vi "estiOptState.vi"(7 "Filter Type":u16(ring) items=["ref", "u", "g", "r", "i", "z", "y"], 8 "error in (no error)":errorcluster, 9 "Field Idx":i32[](array[numeric]), 10 "Zk":dbl[][](array[numeric]), 11 "OptStateEsti in":refnum<class "OptStateEsti.lvclass">) -> (0 "error out":errorcluster, 2 "Optical State":dbl[](array[numeric]), 3 "OptStateEsti out":refnum<class "OptStateEsti.lvclass">)   [LabVIEW 2016, in "OptStateEsti.lvclass"]
doc: "Estimate the optical state in the basis of degree of freedom (DOF)."
uses:
  OptStateEsti.lvclass
  OptStateEsti.lvclass/OptStateEsti.ctl
  <vilib>/Analysis/baseanly.llb/Real A x B.vi
  Utility/getSubArray2D.vi
  <vilib>/Analysis/Matrix/Numeric/Conversions/Array To Matrix - RA2.vi
  <vilib>/Analysis/Matrix/Numeric/Conversions/Matrix To Array - RM.vi
  <vilib>/Analysis/Matrix/NI_Matrix.lvlib
  <vilib>/Analysis/NI_AALBase.lvlib
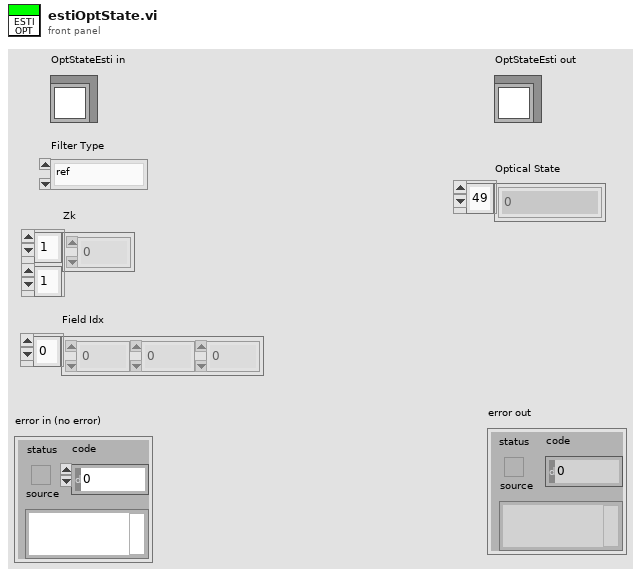
[diagram p1: front panel]
types:
  T1 = typedef "NI_Matrix.lvlib/RealMatrix.ctl" = dbl[][]
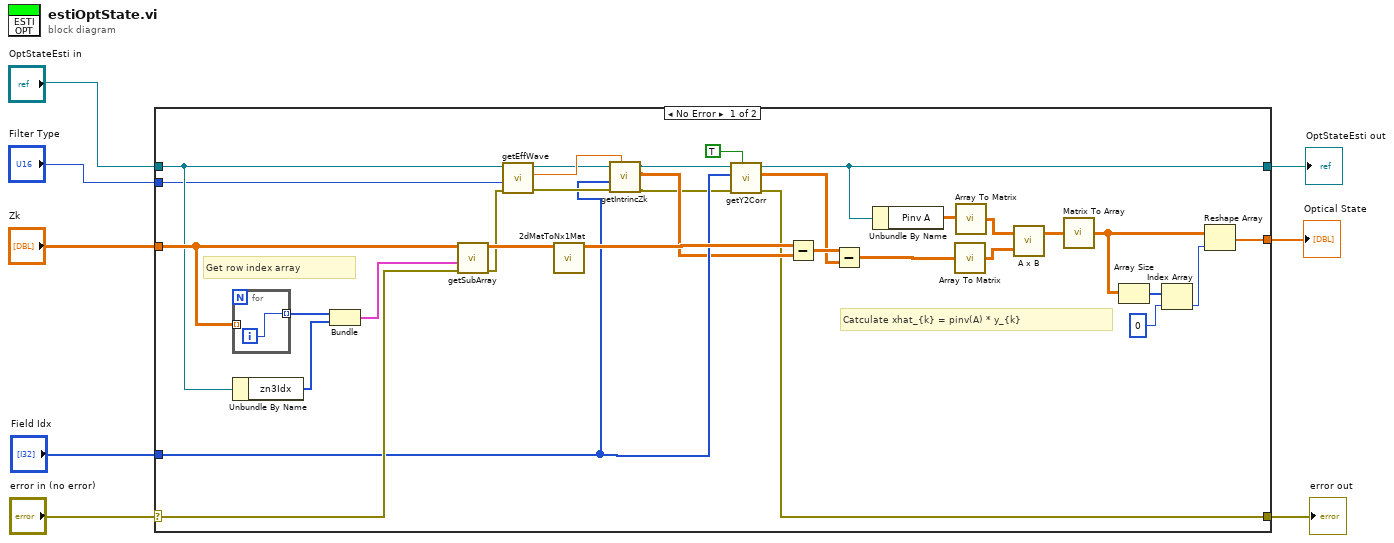
[diagram p0: block diagram]
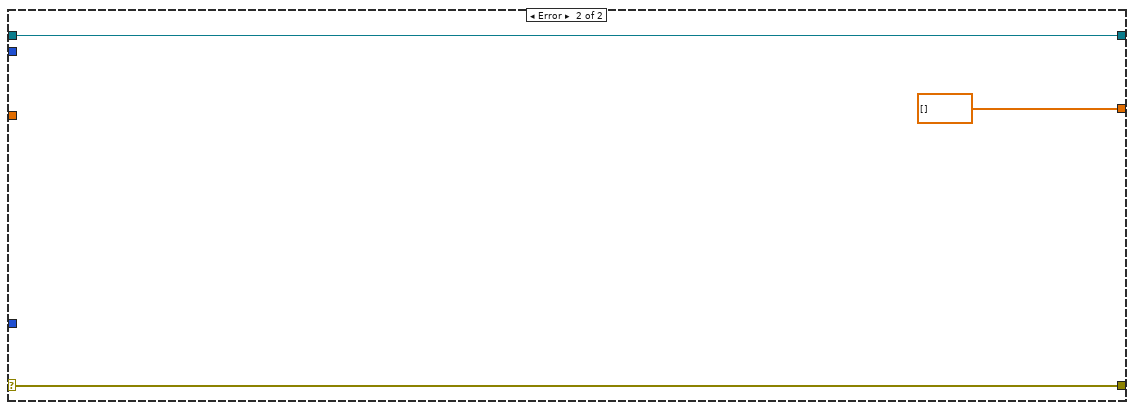
[diagram p2: hidden frame]
diagram:
  n1 = case shown="No Error" "error in (no error)" {
    selector: "error in (no error)" -> [w23 w44]
    tunnel: [w10 w44] -> w7
    tunnel: [w11 w43] -> w6
    tunnel: "OptStateEsti in" -> [w22 w43]
    tunnel: "Zk" -> [w26 _]
    tunnel: "Field Idx" -> [w16 _]
    tunnel: [w29 dbl[] [] ("Real 2D Array")] -> w3
    tunnel: "Filter Type" -> [w21 _]
    frame No Error {
      # "Catculate xhat_{k} = pinv(A) * y_{k}"
      # "Get row index array"
      n2 = for {
        tunnel: w26 -> [_] mode=indexing
        tunnel: [w41] -> w28 mode=indexing
        i -> [w41]
      }
      n3 = Unbundle By Name(w22) -> ("zn3Idx"=w27:i32[])
      n4 = Bundle(w28, "zn3Idx"=w27) -> (w25:cluster{i32[], "zn3Idx":i32[]})  [unwired: 1 in]
      n5 = call-poly "getSubArray.vi"("error in (no error)"=w23, "Index Array Cluster"=w25, "2D Array"=w26) -> ("error out"=w20:errorcluster, "Sub-Array"=w24:dbl[][])  [unwired: 7 in]
      n6 = call "getEffWave.vi"("error in (no error)"=w20, "Filter Type"=w21, "OptStateEsti in"=w22) -> ("error out"=w17:errorcluster, "Effective Wavelength  (um)"=w19:dbl, "OptStateEsti out"=w18:refnum<class "OptStateEsti.lvclass">)  [unwired: 6 in]
      n7 = call "2dMatToNx1Mat.vi"("2D Array"=w24) -> ("nx1 Array"=w39:dbl[][])  [unwired: 10 in]
      n8 = call "getIntrincZk.vi"("Effective Wavelength  (um)"=w19, "error in (no error)"=w17, "Field Idx"=w16, "OptStateEsti in"=w18) -> ("error out"=w13:errorcluster, "Intrinsic Zk"=w14:dbl[][], "OptStateEsti out"=w15:refnum<class "OptStateEsti.lvclass">)  [unwired: 5 in]
      n9 = call "getY2Corr.vi"("In nx1 Row"=TRUE, "error in (no error)"=w13, "Field Idx"=w16, "OptStateEsti in"=w15) -> ("error out"=w10:errorcluster, "y2c Array"=w38:dbl[][], "OptStateEsti out"=w11:refnum<class "OptStateEsti.lvclass">)  [unwired: 5 in]
      n10 = Subtract(x=w39, y=w14) -> (x-y=w40:dbl[][])
      n11 = Subtract(x=w40, y=w38) -> (x-y=w37:dbl[][])
      n12 = Unbundle By Name(w11) -> ("Pinv A"=w12:dbl[][])
      n13 = call-poly <vilib>:"Array To Matrix.vi"("Real 2D Array"=w37) -> ("Real Matrix"=w35:T1)
      n14 = call-poly <vilib>:"Array To Matrix.vi"("Real 2D Array"=w12) -> ("Real Matrix"=w36:T1)
      n15 = call-poly <vilib>:"A x B.vi"("B"=w35, "A"=w36) -> ("A x B"=w34:T1)  [unwired: 1 out]
      n16 = call-poly <vilib>:"Matrix To Array.vi"("Real Matrix"=w34) -> ("Real 2D Array"=w30:dbl[][])
      n17 = Array Size(array=w30) -> (size(s)=w33:i32[])
      n18 = Index Array(array=w33, index=0 ("dimension size")) -> (element=w31:i32)
      n19 = Reshape Array(w30, w31) -> (w29:dbl[])
    }
    frame Error {
    }
  }
  "error out" <- w7
  "OptStateEsti out" <- w6
  "Optical State" <- w3
